vi "Square loop.vi"() -> ()   [LabVIEW 2018]
panel:
  out "Waveform Graph":dbl[](graph)
  out "Intensity Graph":dbl[][](graph)
  in  "Current":dbl
  in  "Length":dbl
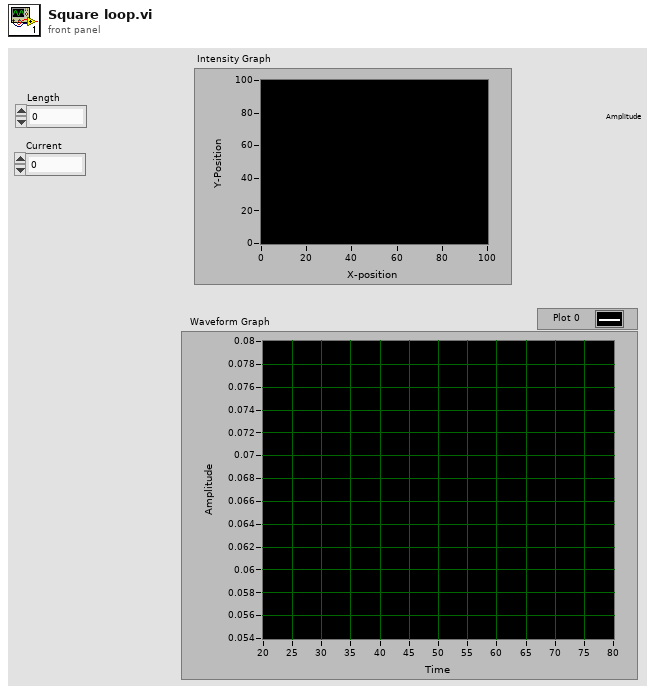
[diagram p1: front panel]
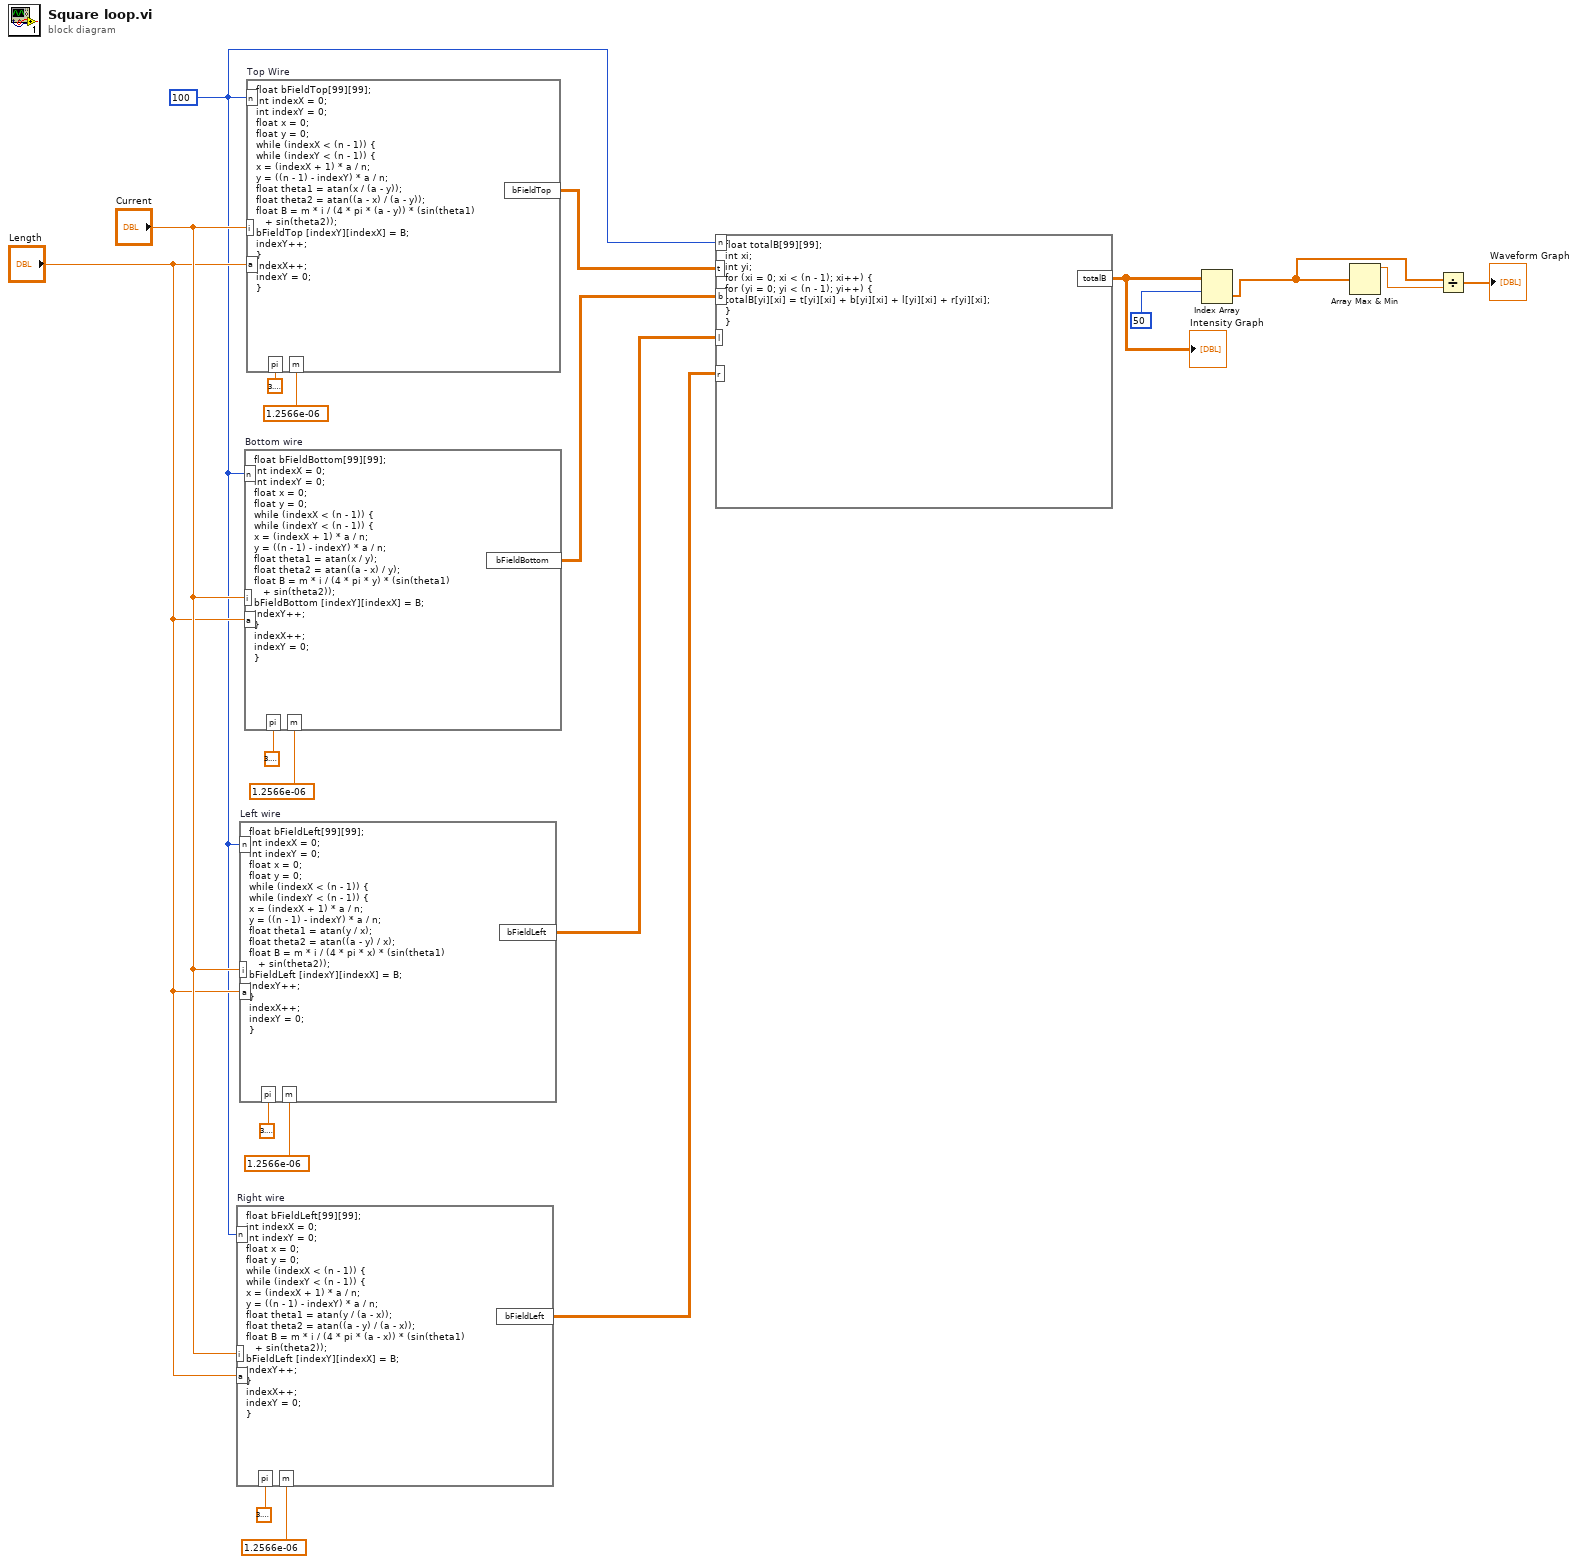
[diagram p0: block diagram]
diagram:
  w6 = 100
  n1 = formula code="float bFieldLeft[99][99];\nint indexX = 0;\nint indexY = 0;\nfloat x = 0;\nfloat y = 0;\nwhile (indexX < (n - 1)) {\nwhile (indexY < (n - 1)) {\nx = (indexX + 1) * a / n;\ny = ((n - 1) - indexY) * a / n;\nfloat theta1 = atan(y / (a - x));\nfloat theta2 = atan((a - y) / (a - x));\nfloat B = m * i / (4 * pi * (a - x)) * (sin(theta1)\n   + sin(theta2));\nbFieldLeft [indexY][indexX] = B;\nindexY++;\n}\nindexX++;\nindexY = 0;\n}" "Right wire"("i"="Current", "a"="Length", "pi"=3.141592653589793, "m"=1.2566e-06, "n"=w6) -> ("bFieldLeft"=w7:dbl[][])
  n2 = formula code="float bFieldLeft[99][99];\nint indexX = 0;\nint indexY = 0;\nfloat x = 0;\nfloat y = 0;\nwhile (indexX < (n - 1)) {\nwhile (indexY < (n - 1)) {\nx = (indexX + 1) * a / n;\ny = ((n - 1) - indexY) * a / n;\nfloat theta1 = atan(y / x);\nfloat theta2 = atan((a - y) / x);\nfloat B = m * i / (4 * pi * x) * (sin(theta1)\n   + sin(theta2));\nbFieldLeft [indexY][indexX] = B;\nindexY++;\n}\nindexX++;\nindexY = 0;\n}" "Left wire"("i"="Current", "a"="Length", "pi"=3.141592653589793, "m"=1.2566e-06, "n"=w6) -> ("bFieldLeft"=w8:dbl[][])
  n3 = formula code="float bFieldBottom[99][99];\nint indexX = 0;\nint indexY = 0;\nfloat x = 0;\nfloat y = 0;\nwhile (indexX < (n - 1)) {\nwhile (indexY < (n - 1)) {\nx = (indexX + 1) * a / n;\ny = ((n - 1) - indexY) * a / n;\nfloat theta1 = atan(x / y);\nfloat theta2 = atan((a - x) / y);\nfloat B = m * i / (4 * pi * y) * (sin(theta1)\n   + sin(theta2));\nbFieldBottom [indexY][indexX] = B;\nindexY++;\n}\nindexX++;\nindexY = 0;\n}" "Bottom wire"("i"="Current", "a"="Length", "pi"=3.141592653589793, "m"=1.2566e-06, "n"=w6) -> ("bFieldBottom"=w9:dbl[][])
  n4 = formula code="float bFieldTop[99][99];\nint indexX = 0;\nint indexY = 0;\nfloat x = 0;\nfloat y = 0;\nwhile (indexX < (n - 1)) {\nwhile (indexY < (n - 1)) {\nx = (indexX + 1) * a / n;\ny = ((n - 1) - indexY) * a / n;\nfloat theta1 = atan(x / (a - y));\nfloat theta2 = atan((a - x) / (a - y));\nfloat B = m * i / (4 * pi * (a - y)) * (sin(theta1)\n   + sin(theta2));\nbFieldTop [indexY][indexX] = B;\nindexY++;\n}\nindexX++;\nindexY = 0;\n}" "Top Wire"("i"="Current", "a"="Length", "pi"=3.141592653589793, "m"=1.2566e-06, "n"=w6) -> ("bFieldTop"=w10:dbl[][])
  n5 = formula code="float totalB[99][99];\nint xi;\nint yi;\nfor (xi = 0; xi < (n - 1); xi++) {\nfor (yi = 0; yi < (n - 1); yi++) {\ntotalB[yi][xi] = t[yi][xi] + b[yi][xi] + l[yi][xi] + r[yi][xi];\n}\n}"("t"=w10, "b"=w9, "l"=w8, "r"=w7, "n"=w6) -> ("totalB"=w5:dbl[][])
  "Intensity Graph" <- w5
  n6 = Index Array(array=w5, index (row)=50) -> (element=w3:dbl[])  [unwired: 1 in]
  n7 = Array Max & Min(array=w3) -> (max value=w2:dbl)  [unwired: 3 out]
  n8 = Divide(x=w3, y=w2) -> (x/y=→"Waveform Graph":dbl[])
